vi "Recorder save.vi"(6 "Set Memory or USB (T:USB F:Memory)":bool, 7 "Channel  (1: CH1)":u16(ring)=1 items=["CH1"=1, "CH2"=2, "CH3"=3, "CH4"=4], 8 "error in (no error)":errorcluster, 9 "Memory(0~9)":u32 max=9, 10 "Name":string, 11 "VISA resource name":refnum<visa-resource-name>) -> (0 "error out":errorcluster, 3 "VISA resource name out":refnum<visa-resource-name>)   [LabVIEW 2020, in "GPP.lvlib"]
uses:
  GPP.lvlib
  Function/VISA_COMMON.ctl
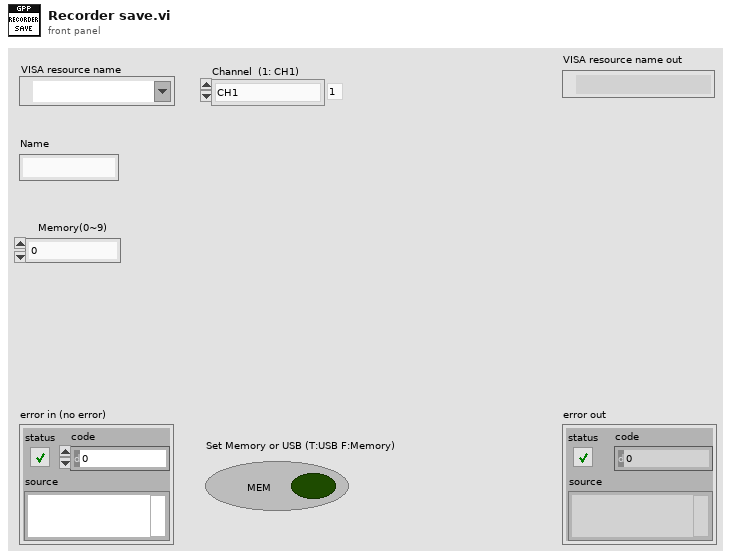
[diagram p1: front panel]
types:
  T1 = typedef "GPP.lvlib/VISA_COMMON.ctl" = enum16{"Initial", "Write CMD", "Read Result", "Read History", "Close"}
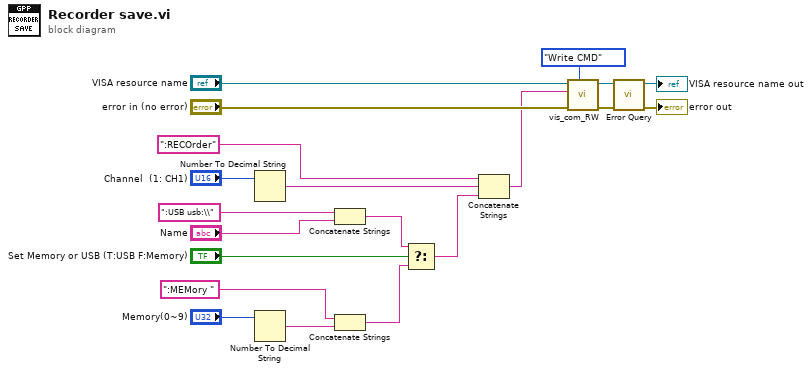
[diagram p0: block diagram]
diagram:
  n1 = Number To Decimal String(number="Channel  (1: CH1)") -> (decimal integer string=w18:string)  [unwired: 1 in]
  n2 = Number To Decimal String(number="Memory(0~9)") -> (decimal integer string=w4:string)  [unwired: 1 in]
  n3 = Concatenate Strings(":USB usb:\\", "Name") -> (w8:string)
  n4 = Concatenate Strings(":MEMory ", w4) -> (w3:string)
  n5 = Select(t=w8, s="Set Memory or USB (T:USB F:Memory)", f=w3) -> (s? t:f=w2:string)
  n6 = Concatenate Strings(":RECOrder", w18, w2) -> (w1:string)
  n7 = call "vis_com_RW.vi"("Funciton"=VISA_COMMON."Write CMD", "error in (no error)"="error in (no error)", "CMD String"=w1, "VISA resource in"="VISA resource name") -> ("error out"=w14:errorcluster, "VISA resource out"=w16:refnum<visa-resource-name>)  [unwired: 5 in, 1 out]
  n8 = call "Error Query.vi"("error in (no error)"=w14, "VISA resource name"=w16) -> ("error out"=→"error out":errorcluster, "VISA resource name out"=→"VISA resource name out":refnum<visa-resource-name>)  [unwired: 6 in, 2 out]
